vi "FF_CircularPath.vi"(8 "error in (no error)":errorcluster, 9 "WristVelocity":dbl[](array[numeric]), 10 "WristPosition":dbl[](array[numeric]), 11 "Force Field Controller in":refnum<class "ForceField.lvclass">) -> (0 "error out":errorcluster, 1 "ClosestPt":dbl[](array[numeric]) format="%.2f", 2 "Force":dbl[](array[numeric]), 3 "Force Field Controller out":refnum<class "ForceField.lvclass">, 4 "ForceComp":dbl[](array[numeric]))   [LabVIEW 2015, in "ForceField.lvclass"]
uses:
  ForceField.lvclass
  ForceField.lvclass/ForceField.ctl
  <vilib>/Analysis/baseanly.llb/A x Vector.vi
  <vilib>/Analysis/_algsub.llb/Real Vector Norm.vi
  <vilib>/Analysis/baseanly.llb/Dot Product.vi
  <vilib>/Analysis/baseanly.llb/Real Dot Product.vi
  SubVis/ThreePts_PlainEqn.vi
  <vilib>/Analysis/7linalg.llb/Solve Linear Equations.vi
  <vilib>/Analysis/7linalg.llb/Solve Linear Equations (single right hand).vi
  <vilib>/Analysis/baseanly.llb/Solve Linear Equations By Cholesky.vi
  <vilib>/Analysis/baseanly.llb/Real Matrix to Compact Array.vi
  <vilib>/Analysis/baseanly.llb/Real Compact Tri-Matrix Linear Eqs.vi
  <vilib>/Analysis/7linalg.llb/Solve Linear Eqs (General).vi
  <vilib>/Analysis/7linalg.llb/Solve Linear Eqs (Gen, single right hand).vi
  <vilib>/Analysis/NI_AALBase.lvlib
  <vilib>/Analysis/NI_AALPro.lvlib
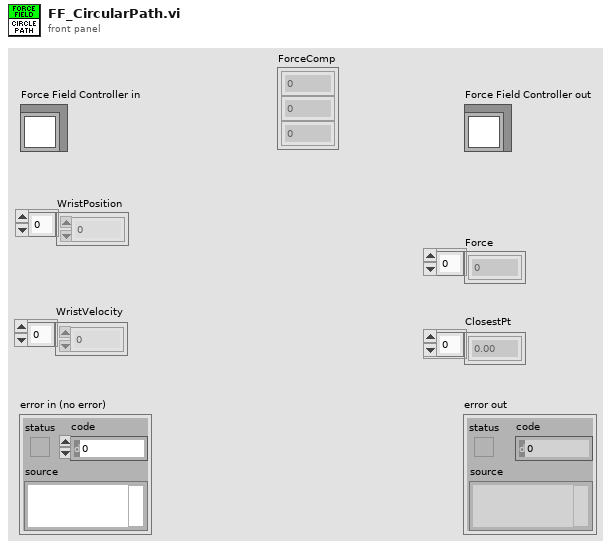
[diagram p1: front panel]
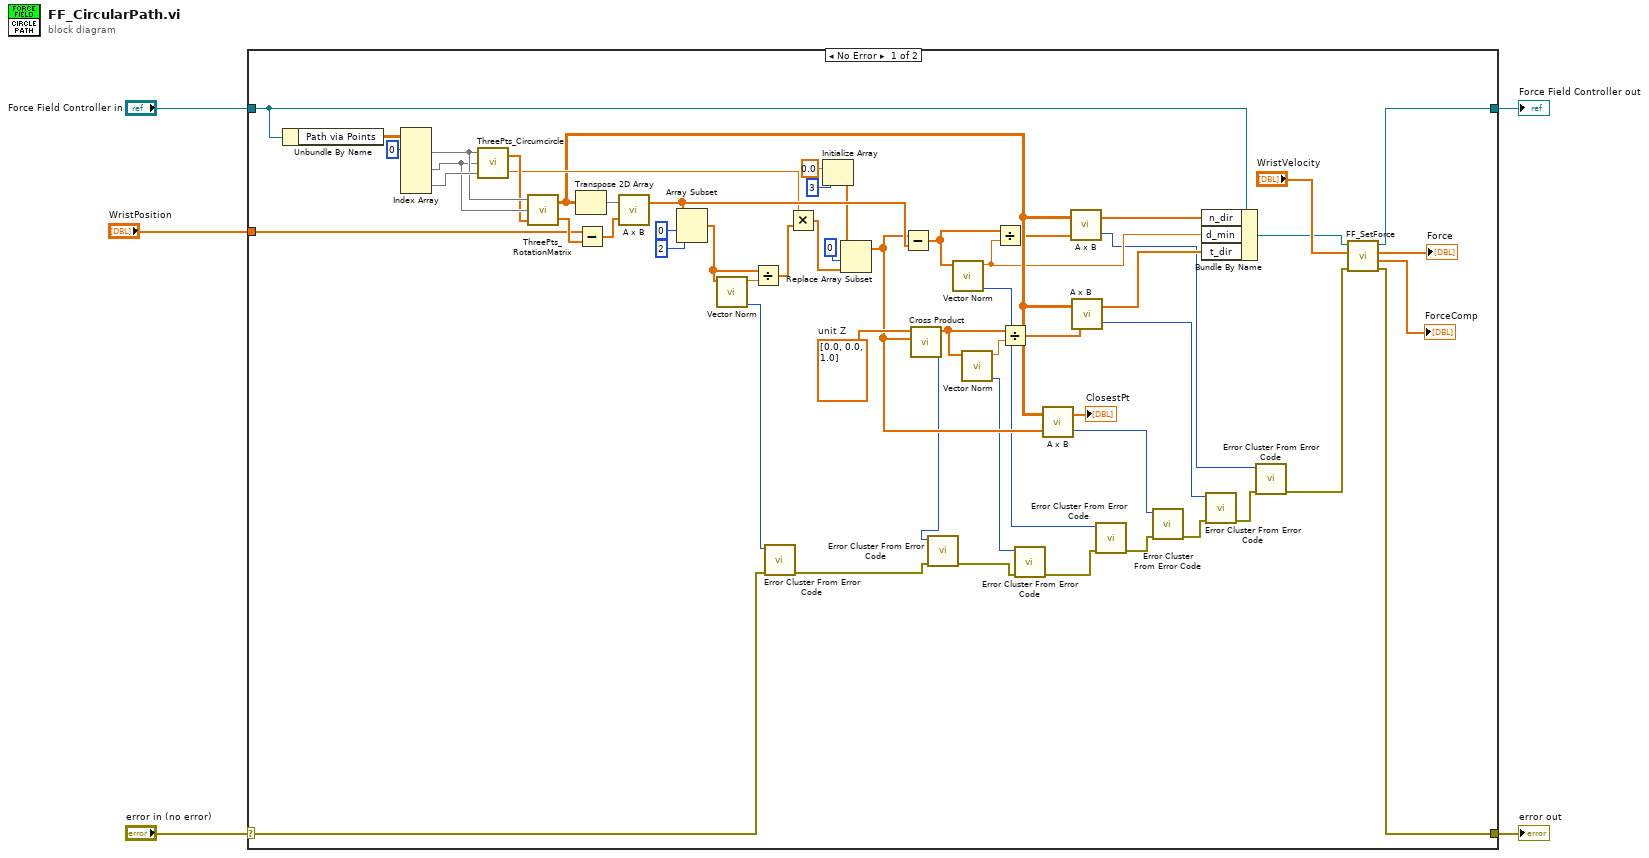
[diagram p0: block diagram]
diagram:
  n1 = case shown="No Error" "error in (no error)" {
    selector: "error in (no error)" -> [w7 w63]
    tunnel: [w34 w63] -> w4
    tunnel: [w35 w62] -> w2
    tunnel: "Force Field Controller in" -> [w39 w62]
    tunnel: "WristPosition" -> [w53 _]
    frame No Error {
      w42 = dbl[] [0.0, 0.0, 1.0]  # unit Z
      n2 = Unbundle By Name(w39) -> ("Path via Points"=w61:dbl[][])
      n3 = Index Array(array=w61, index (row) #1=0 ("index (row)")) -> (element #1=w58:dbl[], element #2=w57:dbl[], element #3=w59:dbl[])  [unwired: 5 in]
      n4 = call "ThreePts_Circumcircle.vi"("V3"=w59, "V2"=w57, "V1"=w58) -> ("Radius"=w48:dbl, "Circumcenter"=w56:dbl[])
      n5 = call "ThreePts_RotationMatrix.vi"("Circumcenter"=w56, "V 2"=w57, "V 1"=w58) -> ("Circumcenter"=w54:dbl[], "Rotation Matrix ( Local to Global )"=w33:dbl[][])
      n6 = Transpose 2D Array(2D array=w33) -> (transposed array=w55:dbl[][])
      n7 = Subtract(x=w53, y=w54) -> (x-y=w52:dbl[])
      n8 = call-poly <vilib>:"A x B.vi"("Vector"=w52, "A"=w55) -> ("A x Vector"=w49:dbl[])  [unwired: 1 out]
      n9 = Array Subset(array=w49, index=0, length=2) -> (w28:dbl[])
      n10 = call-poly <vilib>:"Vector Norm.vi"("Input Vector"=w28) -> ("error"=w26:i32, "norm"=w29:dbl)  [unwired: 9 in]
      n11 = Divide(x=w28, y=w29) -> (x/y=w27:dbl[])
      n12 = call <vilib>:"Error Cluster From Error Code.vi"("error in (no error)"=w7, "error code (0)"=w26) -> ("error out"=w8:errorcluster)  [unwired: 7 in]
      n13 = Multiply(x=w48, y=w27) -> (x*y=w43:dbl[])
      n14 = Initialize Array(0.0 ("element"), 3 ("dimension size")) -> (w45:dbl[])
      n15 = Replace Array Subset(array=w45, new element=w43, index=0) -> (w32:dbl[])
      n16 = Subtract(x=w32, y=w49) -> (x-y=w25:dbl[])
      n17 = call <vilib>:"Cross Product.vi"("B Vector"=w32, "A Vector"=w42) -> ("error"=w9:i32, "Cross Product"=w20:dbl[])  [unwired: 8 in]
      n18 = call <vilib>:"Error Cluster From Error Code.vi"("error in (no error)"=w8, "error code (0)"=w9) -> ("error out"=w10:errorcluster)  [unwired: 7 in]
      n19 = call-poly <vilib>:"Vector Norm.vi"("Input Vector"=w25) -> ("error"=w11:i32, "norm"=w24:dbl)  [unwired: 9 in]
      n20 = call-poly <vilib>:"Vector Norm.vi"("Input Vector"=w20) -> ("error"=w19:i32, "norm"=w21:dbl)  [unwired: 9 in]
      n21 = Divide(x=w25, y=w24) -> (x/y=w23:dbl[])
      n22 = Divide(x=w20, y=w21) -> (x/y=w22:dbl[])
      n23 = call <vilib>:"Error Cluster From Error Code.vi"("error in (no error)"=w10, "error code (0)"=w19) -> ("error out"=w12:errorcluster)  [unwired: 7 in]
      n24 = call-poly <vilib>:"A x B.vi"("Vector"=w32, "A"=w33) -> ("error"=w18:i32, "A x Vector"=→"ClosestPt":dbl[])
      n25 = call-poly <vilib>:"A x B.vi"("Vector"=w23, "A"=w33) -> ("error"=w16:i32, "A x Vector"=w41:dbl[])
      n26 = call-poly <vilib>:"A x B.vi"("Vector"=w22, "A"=w33) -> ("error"=w17:i32, "A x Vector"=w40:dbl[])
      n27 = call <vilib>:"Error Cluster From Error Code.vi"("error in (no error)"=w12, "error code (0)"=w11) -> ("error out"=w13:errorcluster)  [unwired: 7 in]
      n28 = call <vilib>:"Error Cluster From Error Code.vi"("error in (no error)"=w13, "error code (0)"=w18) -> ("error out"=w14:errorcluster)  [unwired: 7 in]
      n29 = Bundle By Name(cluster=w39, "n_dir"=w41, "d_min"=w24, "t_dir"=w40) -> (w36:refnum<class "ForceField.lvclass">)
      n30 = call <vilib>:"Error Cluster From Error Code.vi"("error in (no error)"=w14, "error code (0)"=w17) -> ("error out"=w15:errorcluster)  [unwired: 7 in]
      n31 = call <vilib>:"Error Cluster From Error Code.vi"("error in (no error)"=w15, "error code (0)"=w16) -> ("error out"=w6:errorcluster)  [unwired: 7 in]
      n32 = call "FF_SetForce.vi"("error in (no error)"=w6, "AnkleVelocity"="WristVelocity", "Force Field Controller in"=w36) -> ("error out"=w34:errorcluster, "ForceNTD"=→"ForceComp":dbl[], "ForceXYZ"=→"Force":dbl[], "Force Field Controller out"=w35:refnum<class "ForceField.lvclass">)  [unwired: 5 in]
    }
    frame Error {
    }
  }
  "error out" <- w4
  "Force Field Controller out" <- w2
